vi "Handle Last Ack Core.vi"(4 "error in (no error)":errorcluster, 6 "Last Ack":refnum<class "Last Ack.lvclass">, 7 "Cobra RT in":refnum<class "Cobra RT.lvclass">) -> (0 "error out":errorcluster, 3 "Cobra RT out":refnum<class "Cobra RT.lvclass">)   [LabVIEW 2019, in "Cobra RT.lvlib" / "Cobra RT.lvclass"]
doc: "(<B>Filename</B>: Actor Framework.lvlib:Actor.lvclass:Handle Last Ack Core.vi)\n\nDefines how the caller actor responds to the Last Ack message from a nested actor. The Last Ack message is the final message a nested actor sends to its caller before it shuts down. The message contains information about the final state of the nested actor.\n\nBy default, this method does nothing except return any error the nested actor sent. A descendant class may override this method to define behavior."
uses:
  Cobra RT.lvclass
  <vilib>/ActorFramework/LastAck/Last Ack.lvclass
  <vilib>/MGI/Panel Manager/Panel Actor/Panel Actor/Panel Actor.lvclass
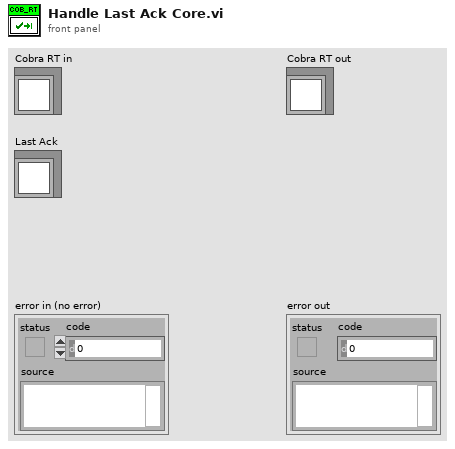
[diagram p1: front panel]
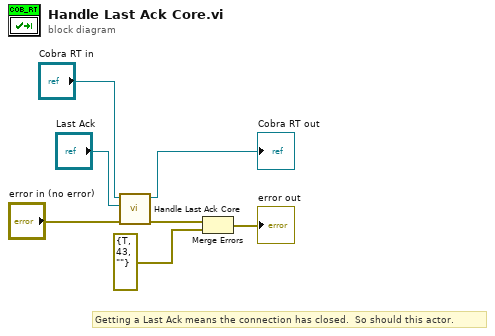
[diagram p0: block diagram]
diagram:
  # "Getting a Last Ack means the connection has closed.  So should this actor."
  n1 = call-parent "Handle Last Ack Core.vi"("error in (no error)"="error in (no error)", "Last Ack"="Last Ack", "Actor in"="Cobra RT in") -> ("error out"=w2:errorcluster, "Actor out"=→"Cobra RT out":refnum<class "Cobra RT.lvclass">)  [unwired: 3 in]
  n2 = Merge Errors(w2, errorcluster {"status"=TRUE, "code"=43, "source"=""} ("error in")) -> (→"error out":errorcluster)
